vi "cleaning_bt.vi"(2 "connection ID in":refnum<k31>) -> (0 "connection ID out":refnum<k31>, 1 "junk buffer":string[](array[string]))   [LabVIEW 2012]
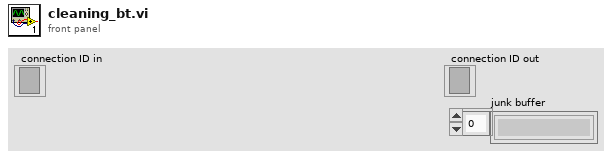
[diagram p1: front panel]
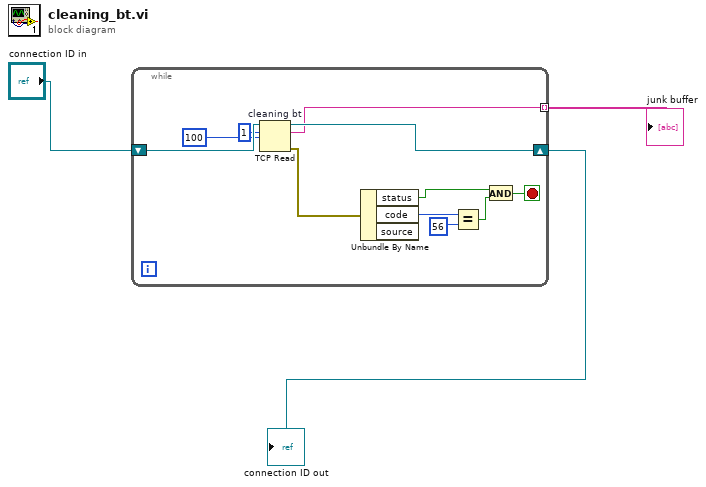
[diagram p0: block diagram]
diagram:
  n1 = while {
    shift-right: [w13] -> w2
    shift-left: "connection ID in" -> [w14]
    tunnel: [w9] -> w3 mode=indexing
    stop <- w6 stop-if-true
    n2 = TCP Read "cleaning bt"(connection ID=w14, bytes to read=1, 9:100 ("timeout ms (25000)")) -> (connection ID out=w13:refnum<k31>, data out=w9:string, error out=w10:errorcluster)  [unwired: 2 in]
    n3 = Unbundle By Name(w10) -> ("status"=w5:bool, "code"=w7:i32)  [unwired: 1 out]
    n4 = Equal?(x=w7, y=u8 56) -> (x = y?=w4:bool)
    n5 = And(x=w5, y=w4) -> (x .and. y?=w6:bool)
  }
  "connection ID out" <- w2
  "junk buffer" <- w3
